vi "ASI_Z_move_serial.vi"(2 "Z position (um)":dbl, 3 "error in":errorcluster, 5 "VISA resource name":refnum<visa-resource-name>) -> (0 "error out":errorcluster, 1 "VISA resource name out":refnum<visa-resource-name>)   [LabVIEW 2018]
panel:
  out "Number of cycles":i32
  out "read buffer after STATUS":string
  out "Number of Bytes at Serial Port":u32
  out "read buffer after MOVE":string
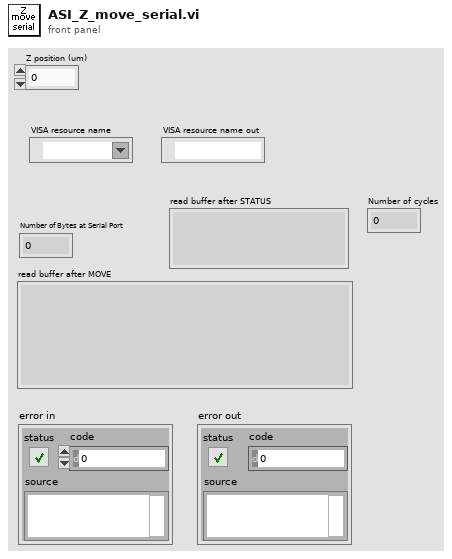
[diagram p1: front panel]
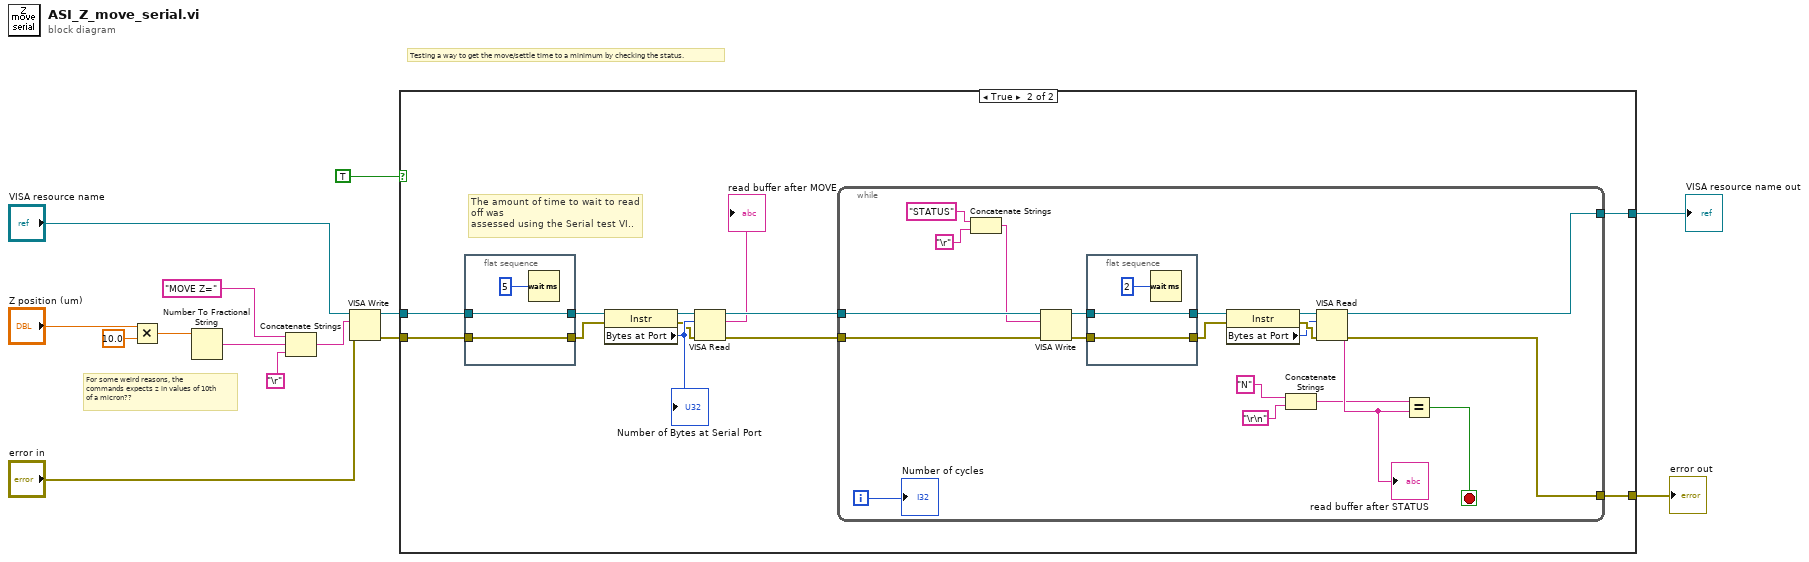
[diagram p0: block diagram]
diagram:
  # "Testing a way to get the move/settle time to a minimum by checking the status."
  # "For some weird reasons, the \ncommands expects z in values of 10th \nof a micron??"
  n1 = Multiply(x="Z position (um)", y=10.0) -> (x*y=w2:dbl)
  n2 = Number To Fractional String(number=w2) -> (F-format string=w4:string)  [unwired: 3 in]
  n3 = Concatenate Strings("MOVE Z=" ("string"), w4, "\r") -> (w14:string)
  n4 = VISA Write(VISA resource name="VISA resource name", write buffer=w14, error in (no error)="error in") -> (VISA resource name out=w13:refnum<visa-resource-name>, error out=w10:errorcluster)  [unwired: 1 out]
  n5 = case shown="True" TRUE {
    tunnel: w13 -> [w16 w28]
    tunnel: w10 -> [w15 w27]
    tunnel: [w15 w23] -> w9
    tunnel: [w16 w24] -> w8
    frame False {
    }
    frame True {
      # "The amount of time to wait to read off was \nassessed using the Serial test VI.."
      n6 = flat-sequence {
        tunnel: [w31] -> w19
        tunnel: w28 -> [w31]
        tunnel: [w29] -> w18
        tunnel: w27 -> [w29]
        frame #0 {
          n7 = Wait (ms)(milliseconds to wait=u32 5) -> ()  [unwired: 1 out]
        }
      }
      n8 = property class="Instr"(reference=w19, error in=w18) -> (reference out=w22:refnum<visa-resource-name>, error out=w17:errorcluster, "Bytes at Port"=w21:u32)
      "Number of Bytes at Serial Port" <- w21
      n9 = VISA Read(VISA resource name=w22, byte count=w21, error in (no error)=w17) -> (VISA resource name out=w26:refnum<visa-resource-name>, read buffer=→"read buffer after MOVE":string, error out=w25:errorcluster)  [unwired: 1 out]
      n10 = while {
        tunnel: w26 -> [w51]
        tunnel: w25 -> [w50]
        tunnel: [w40] -> w24
        tunnel: [w39] -> w23
        i -> [w32]
        stop <- w41 stop-if-true
        n11 = Concatenate Strings("STATUS" ("write buffer"), "\r") -> (w34:string)
        n12 = VISA Write(VISA resource name=w51, write buffer=w34, error in (no error)=w50) -> (VISA resource name out=w44:refnum<visa-resource-name>, error out=w43:errorcluster)  [unwired: 1 out]
        n13 = flat-sequence {
          tunnel: [w54] -> w47
          tunnel: w44 -> [w54]
          tunnel: [w52] -> w48
          tunnel: w43 -> [w52]
          frame #0 {
            n14 = Wait (ms)(milliseconds to wait=u32 2) -> ()  [unwired: 1 out]
          }
        }
        n15 = property class="Instr"(reference=w47, error in=w48) -> (reference out=w45:refnum<visa-resource-name>, error out=w49:errorcluster, "Bytes at Port"=w46:u32)
        n16 = Concatenate Strings("N" ("x"), "\r\n") -> (w37:string)
        n17 = VISA Read(VISA resource name=w45, byte count=w46, error in (no error)=w49) -> (VISA resource name out=w40:refnum<visa-resource-name>, read buffer=w42:string, error out=w39:errorcluster)  [unwired: 1 out]
        "read buffer after STATUS" <- w42
        n18 = Equal?(x=w37, y=w42) -> (x = y?=w41:bool)
        "Number of cycles" <- w32
      }
    }
  }
  "error out" <- w9
  "VISA resource name out" <- w8
